vi "Queue Comms Dequeue.vi"(8 "error in (no error)":errorcluster) -> (0 "error out":errorcluster, 2 "# elements in queue":i32, 3 "element":T1)   [LabVIEW 2018, in "PC UDP Writer.lvlib"]
doc: "This subVI dequeues an element from the communications queue using the Queue Comms FGV"
uses:
  PC UDP Writer.lvlib
  Private Controls/Module Data.ctl
  Private Controls/Module Action.ctl
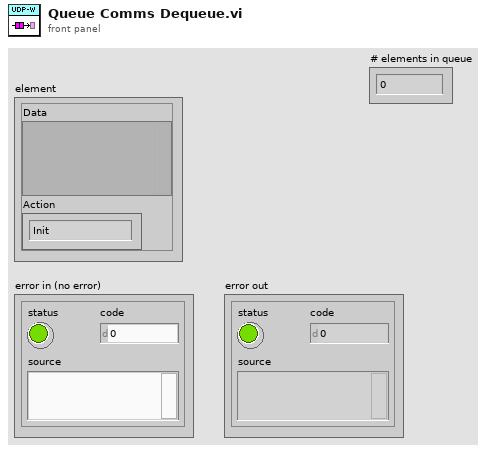
[diagram p1: front panel]
types:
  T1 = typedef "PC UDP Writer.lvlib/Module Data.ctl" = cluster{"Data":variant, "Action":T2}
  T2 = typedef "PC UDP Writer.lvlib/Module Action.ctl" = enum8{"Init", "Waterfall Select", "Bleed Fuel", "Fuel Pressure Reg", "ECS Demand", "Accel Sensitivities", "Accel Filters", "Shunt Relay", "APU Setup", "APU and ECU Control", "APU Start", "Write", "Error", "Exit"}
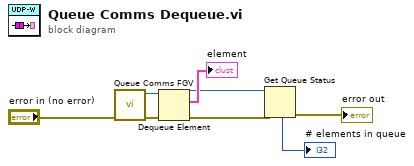
[diagram p0: block diagram]
diagram:
  n1 = call "Queue Comms FGV.vi"("error in (no error)"="error in (no error)") -> ("error out"=w7:errorcluster, "Queue out"=w6:refnum<queue>)  [unwired: 9 in]
  n2 = Dequeue Element(queue=w6, error in (no error)=w7) -> (queue out=w3:refnum<queue>, element=→"element":T1, error out=w4:errorcluster)  [unwired: 1 in, 1 out]
  n3 = Get Queue Status(queue=w3, error in (no error)=w4) -> (error out=→"error out":errorcluster, # elements in queue=→"# elements in queue":i32)  [unwired: 1 in, 6 out]
